vi "Circle Buffer Example.vi"() -> ()   [LabVIEW 2017]
uses:
  <vilib>/measure/matone.llb/Extract Single Tone Information 1 Chan.vi
  <vilib>/measure/NI_MABase.lvlib
  <vilib>/measure/NI_MAPro.lvlib
panel:
  out "Waveform Graph":dbl[](graph)
  out "Waveform Chart":dbl(graph)
  in  "stop":bool
  out "detected frequency":dbl format="%.2p"
  in  "frequency":dbl(slide)=10.0 scale=2.0..50.0
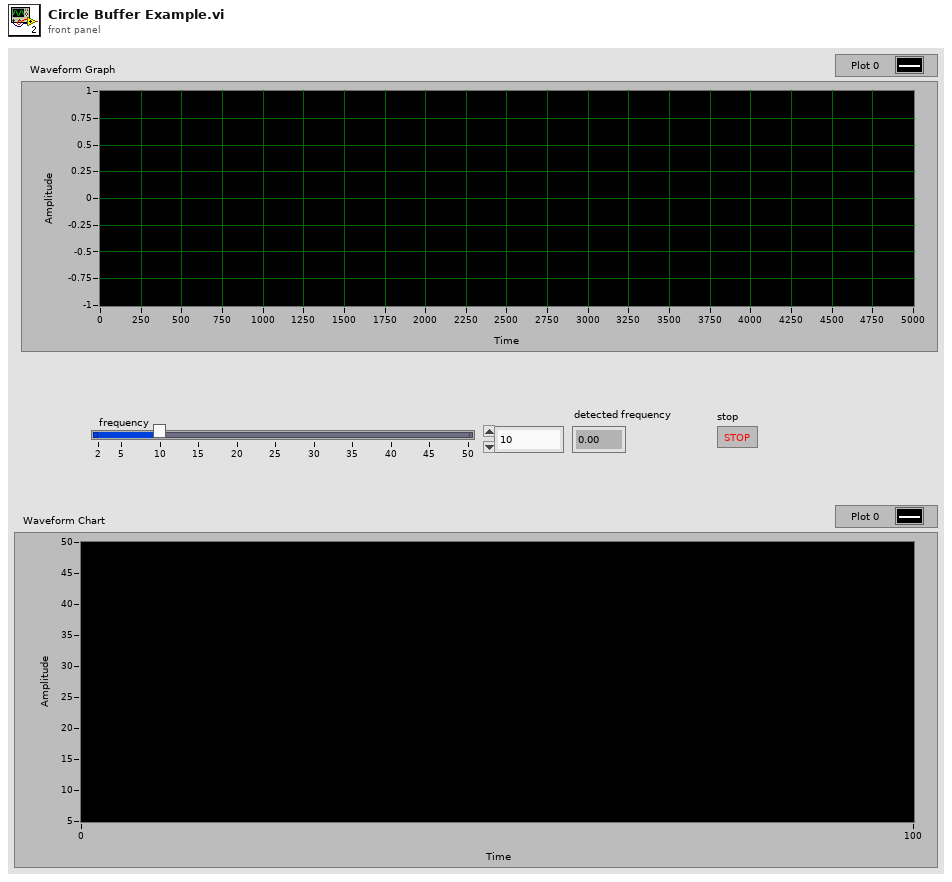
[diagram p1: front panel]
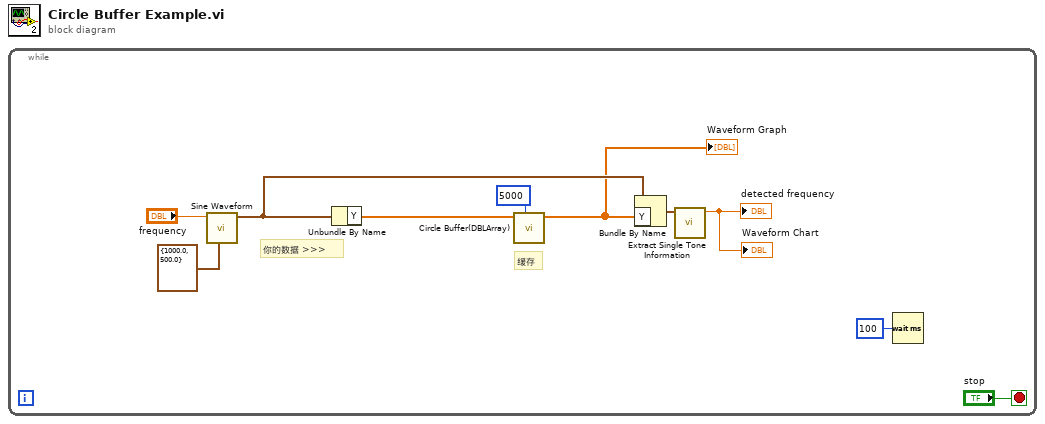
[diagram p0: block diagram]
diagram:
  n1 = while {
    stop <- "stop" stop-if-true
    # "缓存"
    # "你的数据 >>>"
    n2 = call <vilib>:"Sine Waveform.vi"("sampling info"=cluster{"Fs":dbl, "#s":dbl} {"Fs"=1000.0, "#s"=500.0}, "frequency"="frequency") -> ("signal out"=w8:waveform(dbl))  [unwired: 8 in, 1 out]
    n3 = Unbundle By Name(w8) -> ("Y"=w9:dbl[])
    n4 = call "Circle Buffer(DBLArray).vi"("#Count"=5000, "Data"=w9) -> ("Array"=w2:dbl[])  [unwired: 7 in]
    "Waveform Graph" <- w2
    n5 = Bundle By Name(cluster=w8, "Y"=w2) -> (w7:waveform(dbl))
    n6 = call-poly <vilib>:"Extract Single Tone Information.vi"("time signal in"=w7) -> ("detected frequency"=→"detected frequency" →"Waveform Chart":dbl)  [unwired: 5 in, 5 out]
    n7 = Wait (ms)(milliseconds to wait=u32 100) -> ()  [unwired: 1 out]
  }
